vi "ICR_Hardware_Setup.vi"(8 "error in (no error)":errorcluster, 10 "Use Software Trigger":bool=TRUE, 11 "QMH UI Cluster":variant) -> (0 "error out":errorcluster, 3 "HARDWARE Resources":T1={"AO6711 Physical Channels"="AnalogOutput/ao0:3", "AWG5421 Resource Name"="WaveformGenerator", "DIGIT 5122 Resource Name"="Digitizer", "HSDIO Resource Name"="SequencerHSDIO"})   [LabVIEW 2015]
doc: "This VI inits a waveform generation session for HSDIO 6541. This is a basic example that shows how to setup the board in order to generate waveforms according to a script. \n\n1. Initialize for a generation session.\n2. Assign specified channels in Channel List for dynamic operation : all = \"\" (default)\n3. Sets the Idle State for when the generation has completed : NO !!\n4. Configure the Sample clock to use the onboard clock, and configure the clock rate.\n5. Set generation mode to Scripted.\n6. Configure the Script Trigger : change to Digital Edge if waiting for an external\n trigger, and link Rising Edge and source trigger commands.\n Use PFI0 with SMB wired to the board, or any PFIxx if connected to accessory."
uses:
  controls/HARDWARE_Resources.ctl
  controls/QMH_UI_Cluster.ctl
  controls/QMH_UI_References.ctl
  controls/QMH_UI_Report.ctl
  controls/QMH_UI_Command.ctl
  controls/QMH_ICR_Command.ctl
  controls/QMH_Status.ctl
  controls/EXPERT_Inputs.ctl
  controls/SOFTWARE_Inputs.ctl
  controls/AO_6711_Inputs.ctl
  controls/AWG_5421_Inputs.ctl
  controls/DIGIT_5122_Inputs.ctl
  <instrlib>/niScope/Controls/niScope trigger source.ctl
  controls/HSDIO_6541_Inputs.ctl
  <instrlib>/niHSDIO/niHSDIO.llb/niHSDIO_ctl Trigger Source Values (Ring).ctl
  controls/SEQUENCE_Inputs.ctl
  controls/TRAPPING_Inputs.ctl
  controls/EXCIT_Inputs.ctl
  controls/DATA_Inputs.ctl
  controls/TIMING_Inputs.ctl
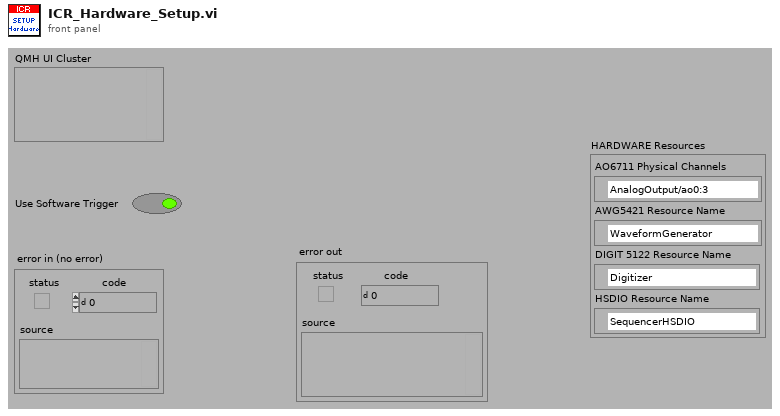
[diagram p1: front panel]
types:
  T1 = typedef "HARDWARE_Resources.ctl" = cluster{"AO6711 Physical Channels":tag, "AWG5421 Resource Name":refnum<k15>, "DIGIT 5122 Resource Name":refnum<k15>, "HSDIO Resource Name":refnum<k15>}
  T2 = typedef "SEQUENCE_Inputs.ctl" = cluster{"TRAPPING Inputs":T3, "EXCIT Inputs":T4, "DATA Inputs":T5, "TIMING Inputs":T6}
  T3 = typedef "TRAPPING_Inputs.ctl" = cluster{"Init Values":dbl[], "Opening Values":dbl[], "Trapping Values":dbl[], "Emptying Values":dbl[], "Adiabatic ON":bool, "Adiabatic Duration":i32, "Adiabatic Waveforms":string[]}
  T4 = typedef "EXCIT_Inputs.ctl" = cluster{"Number of Excitations":i32, "Table of Waveforms":string[], "Script text":string}
  T5 = typedef "DATA_Inputs.ctl" = cluster{"Record Length":i32, "Sample Rate":enum16{"1", "2", "5", "10", "20", "25", "50", "100"}, "Number of Acquisitions":i32, "Type Of Data":enum16{"I16", "DBL"}, "Vertical Range":enum16{"0.2", "0.4", "1", "2", "4", "10"}}
  T6 = typedef "TIMING_Inputs.ctl" = cluster{"Number Of Acquisitions ":i16, "Number Of Accumulations":i16, "Number Of Loops":i16, "Table of Waveforms":string[], "Script text":string}
  T7 = typedef "EXPERT_Inputs.ctl" = cluster{"SOFTWARE Inputs":T8, "AO 6711 Inputs":T9, "AWG 5421 Inputs":T10, "DIGIT 5122 Inputs":T11, "HSDIO 6541 Inputs":T13}
  T8 = typedef "SOFTWARE_Inputs.ctl" = cluster{"Application Directory":path, "Resources Path":path, "Data Path":path, "XML Path":path, "XML File Filter":string, "Excit Scripts Path":path, "Excit Scripts File Filter":string, "Excit Waveforms Path":path, "Excit Waveforms File Filter":string, "Timing Scripts Path":path, "Timing Scripts File Filter":string, "Timing Waveforms Path":path, "Timing Waveforms File Filter":string, "Trapping Waveforms Path":path, "Trapping Waveforms File Filter":string}
  T9 = typedef "AO_6711_Inputs.ctl" = cluster{"Physical Channels":tag, "Min Voltage":dbl, "Max Voltage":dbl, "Trigger Source":tag, "counter":tag}
  T10 = typedef "AWG_5421_Inputs.ctl" = cluster{"Resource Name":refnum<k15>, "Trigger Type":u16, "Trigger Source":string, "Sample Rate":dbl}
  T11 = typedef "DIGIT_5122_Inputs.ctl" = cluster{"Sample Rate":dbl, "Resource Name":refnum<k15>, "Channel Name":string, "Trigger Source":T12, "Vertical Range":dbl, "Trigger Level":dbl}
  T12 = typedef "niScope trigger source.ctl" = string
  T13 = typedef "HSDIO_6541_Inputs.ctl" = cluster{"Resource Name":refnum<k15>, "Clock Rate":dbl, "Trigger Source":T14}
  T14 = typedef "niHSDIO_ctl Trigger Source Values (Ring).ctl" = string
  T15 = typedef "QMH_UI_Cluster.ctl" = cluster{"QMH UI References":T16, "QMH UI Report":T17}
  T16 = typedef "QMH_UI_References.ctl" = cluster{"Refnum Load":refnum<vi>, "Refnum Save":refnum<vi>, "Refnum Start":refnum<vi>, "Refnum Stop":refnum<vi>, "Refnum Exit":refnum<vi>, "Refnum Tabs":refnum<vi>, "Refnum SPECTRUM":refnum<vi>, "Refnum EXPERIMENT":refnum<vi>, "Refnum VOLTAGES":refnum<vi>, "Refnum SEQUENCE":refnum<vi>, "Refnum EXPERT":refnum<vi>, "Refnum CHANGE Experiment":refnum<vi>, "Refnum CHANGE Voltages":refnum<vi>, "Refnum CHANGE Sequence":refnum<vi>, "Refnum CHANGE Expert":refnum<vi>}
  T17 = typedef "QMH_UI_Report.ctl" = cluster{"UI Status":T18, "QLA Status":string, "ICR Status":T19, "QMH Status":T20}
  T18 = typedef "QMH_UI_Command.ctl" = enum16{"Initialize", "UI Load", "UI Save", "UI Change Experiment", "UI Change Voltages", "UI Change Sequence", "UI Change Expert", "Ready to Start", "UI Start", "UI Stop", "UI Exit", "Update Report", "Update ICR Report"}
  T19 = typedef "QMH_ICR_Command.ctl" = enum16{"Initialize", "Hardware Setup", "Waiting for Trigger", "Sequence Started", "Sequence Finished", "Writing Data", "Hardware Reset", "Exit"}
  T20 = typedef "QMH_Status.ctl" = enum16{"Init", "Loading", "Setup", "Ready to Start", "Started", "Idle"}
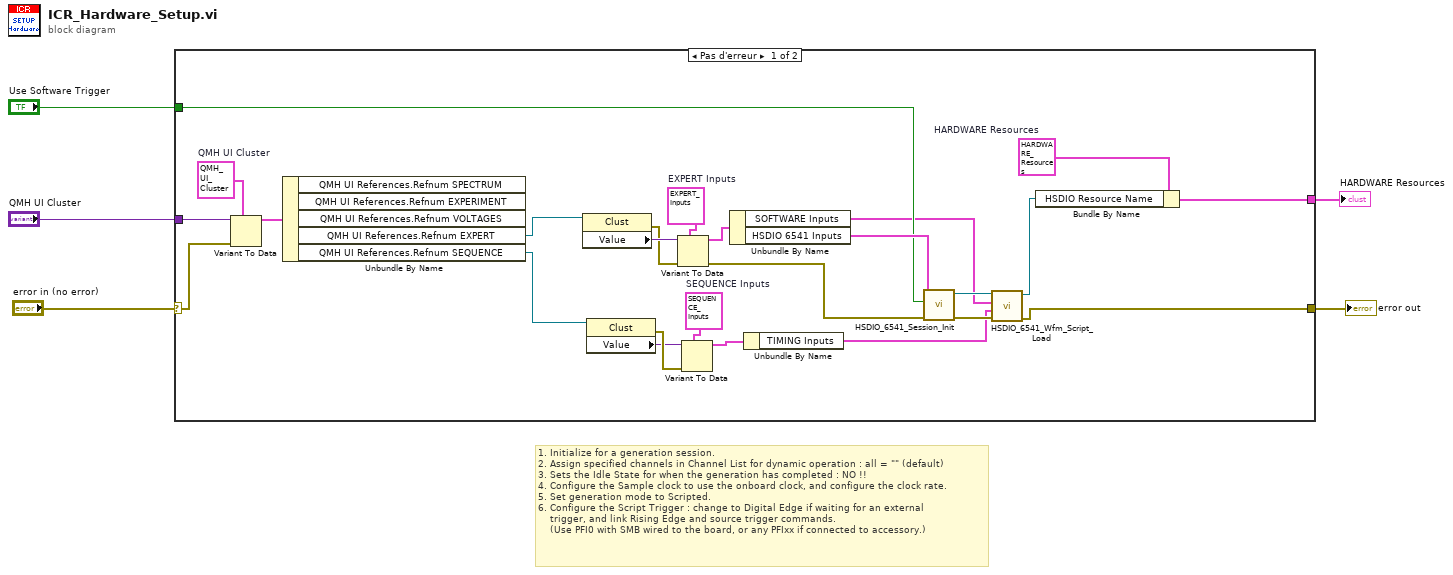
[diagram p0: block diagram]
diagram:
  # "1. Initialize for a generation session.\n2. Assign specified channels in Channel List for dynamic operation : all = \"\" (default)\n3. Sets the Idle State for when the generation has completed : NO !!\n4. Configure the Sample clock to use the onboard clock, and configure the clock rate.\n5. Set generation mode to Scripted.\n6. Configure the Script Trigger : change to Digital Edge if waiting for an external\n    trigger, and link Rising Edge and source trigger commands.\n    (Use PFI0 with SMB wired to the board, or any PFIxx if connected to accessory.)"
  n1 = case shown="Pas d'erreur" "error in (no error)" {
    selector: "error in (no error)" -> [w23 w31]
    tunnel: [w7 w31] -> w5
    tunnel: "Use Software Trigger" -> [w19 _]
    tunnel: "QMH UI Cluster" -> [w30 _]
    tunnel: [w20 _] -> w1
    frame No Error {
      w15 = T2 {"TRAPPING Inputs"={"Init Values"=[2.0, 5.0, 5.0, 2.0], "Opening Values"=[0.0, 0.0, 0.0, 0.0], "Trapping Values"=[2.0, 5.0, 5.0, 2.0], "Emptying Values"=[-5.0, -5.0, -5.0, -5.0], "Adiabatic ON"=FALSE, "Adiabatic Duration"=0, "Adiabatic Waveforms"=["Adiabatic_None_2_2_2000.bin", "Adiabatic_Ramp_5_0_2000.bin", "Adiabatic_DoubleRamp_5_0_2000.bin", "Adiabatic_RC_2_0_2000.bin"]}, "EXCIT Inputs"={"Number of Excitations"=1, "Table of Waveforms"=[], "Script text"=""}, "DATA Inputs"={"Record Length"=8192, "Sample Rate"=enum."5", "Number of Acquisitions"=1, "Type Of Data"=enum."DBL", "Vertical Range"=enum."0.2"}, "TIMING Inputs"={"Number Of Acquisitions "=32767, "Number Of Accumulations"=1, "Number Of Loops"=0, "Table of Waveforms"=[], "Script text"=""}}  # SEQUENCE Inputs
      w21 = T1 {"AO6711 Physical Channels"="AnalogOutput/ao0:3", "AWG5421 Resource Name"="WaveformGenerator", "DIGIT 5122 Resource Name"="Digitizer", "HSDIO Resource Name"="SequencerHSDIO"}  # HARDWARE Resources
      w25 = T7 {"SOFTWARE Inputs"={"Application Directory"=path "D:/S.O.F.T.S/LABVIEW/PIL", "Resources Path"=path "D:/S.O.F.T.S/LABVIEW/PIL/resources", "Data Path"=path "D:/PIRENEA/DATA", "XML Path"=path "D:/PIRENEA/DATA", "XML File Filter"="*.xml", "Excit Scripts Path"=path "D:/PIRENEA/EXCIT_SCRIPTS", "Excit Scripts File Filter"="*.txt", "Excit Waveforms Path"=path "D:/PIRENEA/EXCIT_WFMS", "Excit Waveforms File Filter"="*.bin", "Timing Scripts Path"=path "D:/PIRENEA/SEQUENCE_SCRIPTS", "Timing Scripts File Filter"="*.txt", "Timing Waveforms Path"=path "D:/PIRENEA/SEQUENCE_WFMS", "Timing Waveforms File Filter"="*.bin", "Trapping Waveforms Path"=path "D:/PIRENEA/TRAPPING_WFMS", "Trapping Waveforms File Filter"="*.bin"}, "AO 6711 Inputs"={"Physical Channels"="AnalogOutput/ao0:3", "Min Voltage"=-10.0, "Max Voltage"=10.0, "Trigger Source"="/AnalogOutput/PFI0", "counter"="AnalogOutput/ctr0"}, "AWG 5421 Inputs"={"Resource Name"="WaveformGenerator", "Trigger Type"=2, "Trigger Source"="PFI0", "Sample Rate"=20000000.0}, "DIGIT 5122 Inputs"={"Sample Rate"=10000000.0, "Resource Name"="Digitizer", "Channel Name"="0", "Trigger Source"="VAL_EXTERNAL", "Vertical Range"=10.0, "Trigger Level"=3.0}, "HSDIO 6541 Inputs"={"Resource Name"="SequencerHSDIO", "Clock Rate"=1000000.0, "Trigger Source"="PFI0"}}  # EXPERT Inputs
      w29 = T15 {"QMH UI References"={"Refnum Load"=refnum, "Refnum Save"=refnum, "Refnum Start"=refnum, "Refnum Stop"=refnum, "Refnum Exit"=refnum, "Refnum Tabs"=refnum, "Refnum SPECTRUM"=refnum, "Refnum EXPERIMENT"=refnum, "Refnum VOLTAGES"=refnum, "Refnum SEQUENCE"=refnum, "Refnum EXPERT"=refnum, "Refnum CHANGE Experiment"=refnum, "Refnum CHANGE Voltages"=refnum, "Refnum CHANGE Sequence"=refnum, "Refnum CHANGE Expert"=refnum}, "QMH UI Report"={"UI Status"=enum."Initialize", "QLA Status"="", "ICR Status"=enum."Initialize", "QMH Status"=enum."Init"}}  # QMH UI Cluster
      n2 = Variant To Data(error in=w23, type=w29, Variant=w30) -> (data=w28:T15)  [unwired: 1 out]
      n3 = Unbundle By Name(w28) -> ("QMH UI References.Refnum EXPERT"=w27:refnum<vi>, "QMH UI References.Refnum SEQUENCE"=w13:refnum<vi>)  [unwired: 3 out]
      n4 = property class="Clust"(reference=w27) -> (error out=w18:errorcluster, "Value"=w26:variant)  [unwired: 1 in, 1 out]
      n5 = property class="Clust"(reference=w13) -> (error out=w17:errorcluster, "Value"=w14:variant)  [unwired: 1 in, 1 out]
      n6 = Variant To Data(error in=w18, type=w25, Variant=w26) -> (data=w24:T7, error out=w8:errorcluster)
      n7 = Variant To Data(error in=w17, type=w15, Variant=w14) -> (data=w16:T2)  [unwired: 1 out]
      n8 = Unbundle By Name(w24) -> ("SOFTWARE Inputs"=w10:T8, "HSDIO 6541 Inputs"=w22:T13)
      n9 = Unbundle By Name(w16) -> ("TIMING Inputs"=w9:T6)
      n10 = call "HSDIO_6541_Session_Init.vi"("error in (no error)"=w8, "Use Software Trigger"=w19, "HSDIO 6541 Inputs"=w22) -> ("error out"=w12:errorcluster, "instrument handle out"=w11:refnum<k15>)  [unwired: 7 in]
      n11 = call "HSDIO_6541_Wfm_Script_Load.vi"("error  in"=w12, "TIMING Inputs"=w9, "SOFTWARE Inputs"=w10, "instrument handle in"=w11) -> ("error out"=w7:errorcluster, "instrument handle out"=w6:refnum<k15>)  [unwired: 5 in, 1 out]
      n12 = Bundle By Name(cluster=w21, "HSDIO Resource Name"=w6) -> (w20:T1)
    }
    frame Error {
    }
  }
  "error out" <- w5
  "HARDWARE Resources" <- w1
